vi "Port config dialog.vi"(8 "error in (no error)":errorcluster, 11 "Comm ports in":T3={"Piezo driver"="COM2", "Cam Session"="", "Arduino"="COM2"}) -> (0 "error out":errorcluster, 3 "Comm ports out":T3={"Piezo driver"="COM2", "Cam Session"="", "Arduino"="COM2"})   [LabVIEW 2020]
uses:
  Controls/Config SM states--typedef.ctl
  <vilib>/vision/driver/NI_Vision_Acquisition_Software.lvlib
  7b095cd5-608e-4c75-912f-b4dce6dcc42e.vi
  <userlib>/_OpenG.lib/error/error.llb/openg_error.lvlib
  <vilib>/userDefined/High Color/IMAQdx.ctl
  Controls/Communication ports ---typedef.ctl
panel:
  out "Image":T1(plugin-control)
  out "Test result":string
  in  "Cancel Button":bool
  in  "OK Button":bool
  in  "Test Ard":bool
  in  "Test driver":bool
  in  "Test cam":bool
  in  "Arduino":refnum<visa-resource-name>="COM5"
  in  "Cam Session":T2="cam0"
  in  "Piezo driver":refnum<visa-resource-name>="UNKNOWN"
  out "Comm ports temp":T3={"Piezo driver"="COM2", "Cam Session"="", "Arduino"="COM2"}
  out "Cancelled?":bool
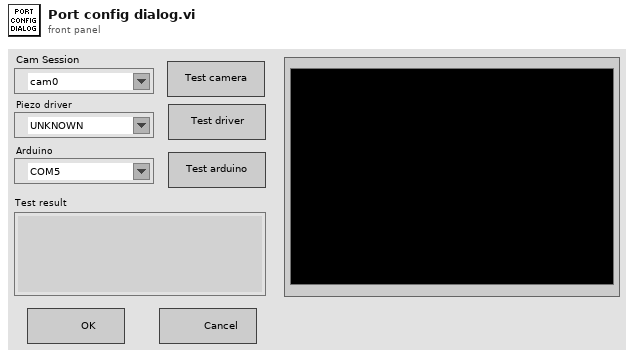
[diagram p1: front panel]
types:
  T1 = typedef "IMAQ Image.ctl" = refnum<image>
  T2 = typedef "IMAQdx.ctl" = refnum<k21>
  T3 = typedef "Communication ports ---typedef.ctl" = cluster{"Piezo driver":refnum<visa-resource-name>, "Cam Session":T2, "Arduino":refnum<visa-resource-name>}
  T4 = typedef "Config SM states--typedef.ctl" = enum16{"Init", "Wait", "Update status", "Accept", "Cancel", "Exit"}
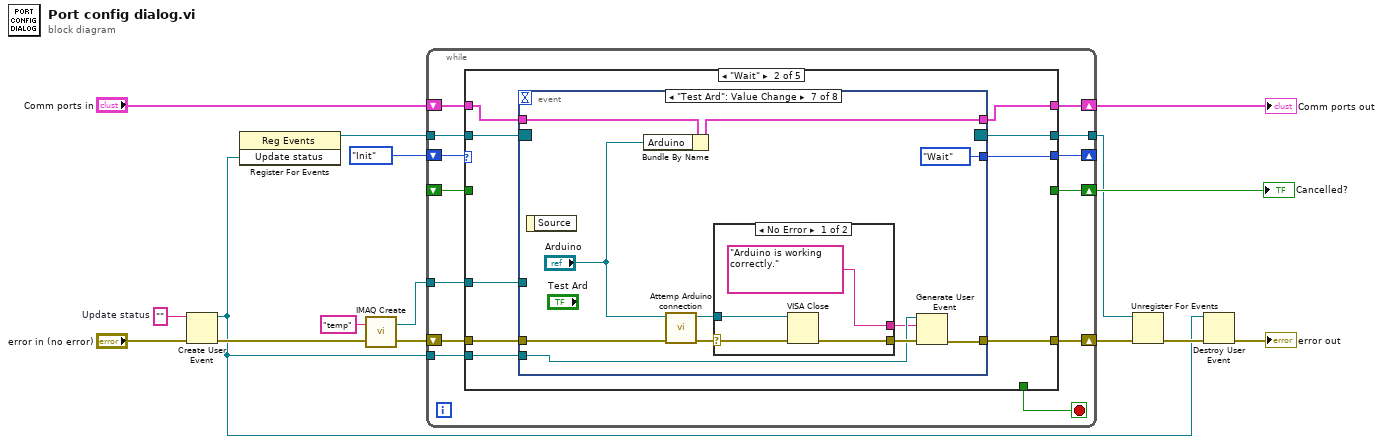
[diagram p0: block diagram]
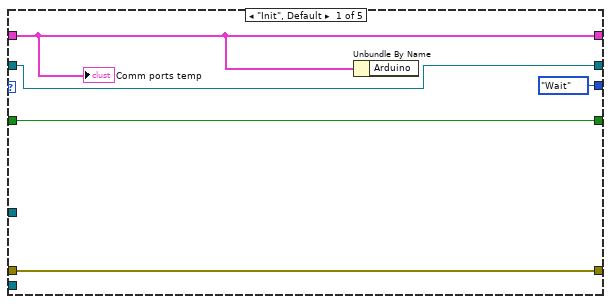
[diagram p2: hidden frame]
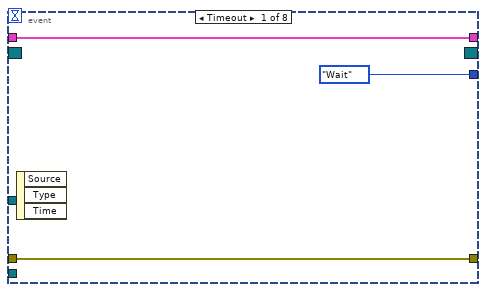
[diagram p3: hidden frame]
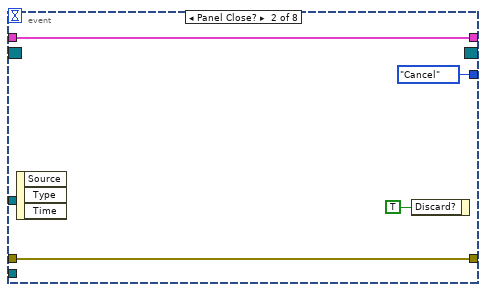
[diagram p4: hidden frame]
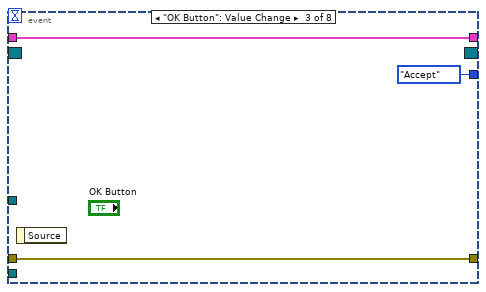
[diagram p5: hidden frame]
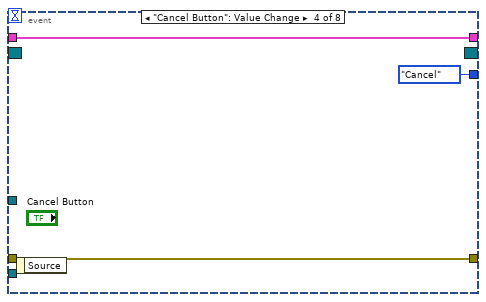
[diagram p6: hidden frame]
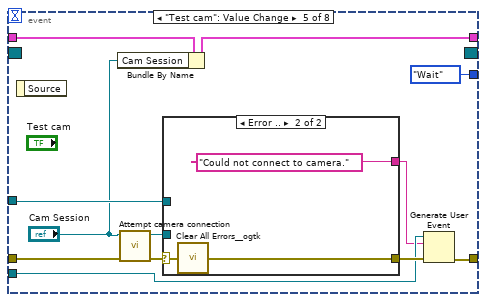
[diagram p7: hidden frame]
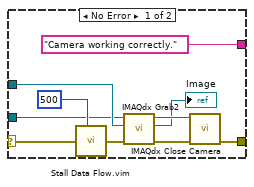
[diagram p8: hidden frame]
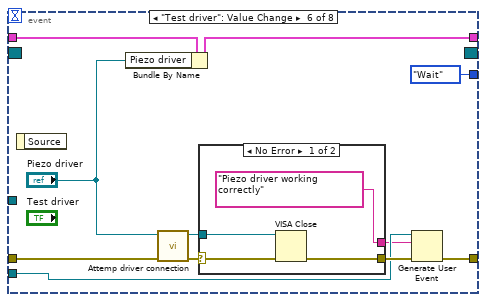
[diagram p9: hidden frame]
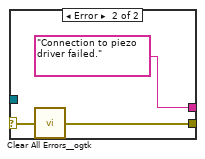
[diagram p10: hidden frame]
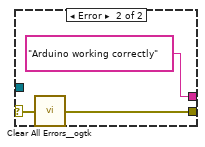
[diagram p11: hidden frame]
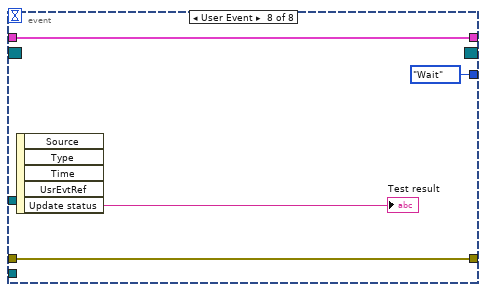
[diagram p12: hidden frame]
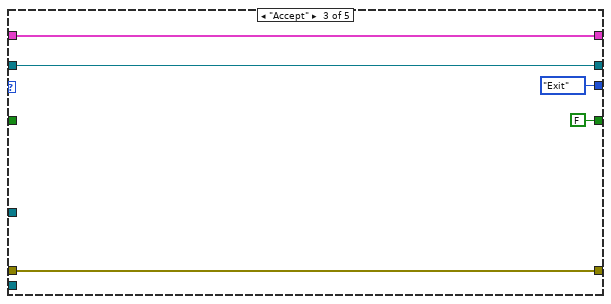
[diagram p13: hidden frame]
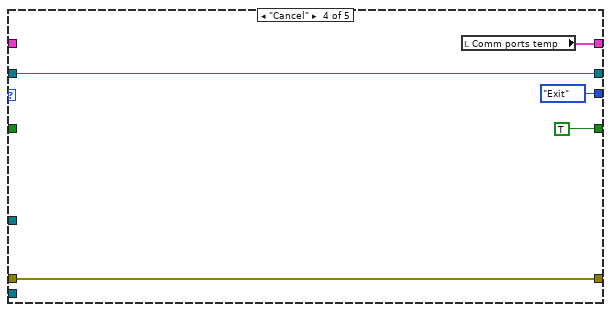
[diagram p14: hidden frame]
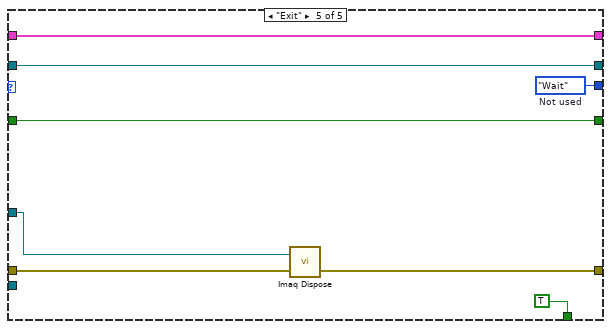
[diagram p15: hidden frame]
diagram:
  w6 = ""  # Update status
  n1 = Create User Event(user event datatype=w6, error in="error in (no error)") -> (user event=w1:refnum<user-event>, error out=w7:errorcluster)
  n2 = register-events(w1) -> (reference out=w5:refnum<event-registration>)  [unwired: 2 in, 1 out]
  n3 = call "IMAQ Create"("Image Name"="temp", "error in (no error)"=w7) -> ("New Image"=w10:T1, "error out"=w8:errorcluster)  [unwired: 3 in]
  n4 = while {
    shift-right: [w24] -> _
    shift-left: Config_SM_states--typedef."Init" -> [w25]
    shift-right: [w22] -> w12
    shift-left: _ -> [w21]
    shift-right: [w28] -> w15
    shift-left: "Comm ports in" -> [w29]
    tunnel: w10 -> [w20]
    shift-right: [w26] -> w14
    shift-left: w8 -> [w27]
    tunnel: w5 -> [w19]
    tunnel: [w18] -> w2
    tunnel: w1 -> [w17]
    stop <- w23 stop-if-true
    n5 = case shown="\"Wait\"" w25 {
      tunnel: w29 -> [w31 w40 w126 _ w139]
      tunnel: [w31 w39 w126 w128 w139] -> w28
      tunnel: w27 -> [w34 w42 w125 w131 w138]
      tunnel: [w34 w41 w125 w131 w135] -> w26
      tunnel: [Config_SM_states--typedef."Wait" w43 Config_SM_states--typedef."Exit" ("Not used") Config_SM_states--typedef."Exit" w137] -> w24
      tunnel: [_ _ _ _ TRUE] -> w23
      tunnel: [w32 _ FALSE TRUE w133] -> w22
      tunnel: w21 -> [w32 _ _ _ w133]
      tunnel: w20 -> [_ w38 _ _ w134]
      tunnel: w19 -> [w30 w37 w122 w127 w132]
      tunnel: [w30 w36 w122 w127 w132] -> w18
      tunnel: w17 -> [_ w35 _ _ _]
      frame "Init", Default {
        n6 = Unbundle By Name(w31) -> ()  [unwired: 1 out]
        "Comm ports temp" <- w31
      }
      frame "Wait" {
        n7 = event shown="[6] \"Test Ard\": Value Change" {
          selector: w37 -> [_ _ _ _ _ _ _ _]
          dyn-events: [_ _ _ _ _ _ _ _] -> w36
          timeout: _ -> [_ _ _ _ _ _ _ _]
          tunnel: [Config_SM_states--typedef."Wait" Config_SM_states--typedef."Cancel" Config_SM_states--typedef."Accept" Config_SM_states--typedef."Cancel" Config_SM_states--typedef."Wait" Config_SM_states--typedef."Wait" Config_SM_states--typedef."Wait" Config_SM_states--typedef."Wait"] -> w43
          tunnel: w42 -> [w45 w48 w53 w56 w64 w92 w108 w121]
          tunnel: [w45 w48 w53 w56 w59 w85 w103 w121] -> w41
          tunnel: w40 -> [w44 w47 w52 w55 w67 w91 w110 w120]
          tunnel: [w44 w47 w52 w55 w66 w89 w109 w120] -> w39
          tunnel: w38 -> [_ _ _ _ w65 _ _ _]
          tunnel: w35 -> [_ _ _ _ w58 w84 w102 _]
          event Timeout {
            n8 = event-data() -> ()  [unwired: 1 in, 3 out]
          }
          event Panel Close? {
            n9 = event-data() -> ()  [unwired: 1 in, 3 out]
            n10 = event-data("Discard?"=TRUE) -> ()  [unwired: 1 in, 1 out]
          }
          event "OK Button": Value Change {
            n11 = event-data() -> ()  [unwired: 1 in, 1 out]
          }
          event "Cancel Button": Value Change {
            n12 = event-data() -> ()  [unwired: 1 in, 1 out]
          }
          event "Test cam": Value Change {
            n13 = event-data() -> ()  [unwired: 1 in, 1 out]
            n14 = Bundle By Name(cluster=w67, "Cam Session"="Cam Session") -> (w66:T3)
            n15 = call "Attempt camera connection.vi"("error in (no error)"=w64, "Camera session"="Cam Session") -> ("error out"=w63:errorcluster, "Cam session Out"=w62:T2)  [unwired: 8 in]
            n16 = case shown="Error .." w63 {
              selector: w63 -> [w71 w80]
              tunnel: [w73 w81] -> w60
              tunnel: w65 -> [w72 _]
              tunnel: w62 -> [w70 _]
              tunnel: ["Camera working correctly." "Could not connect to camera."] -> w57
              frame No Error {
                n17 = call "Stall Data Flow.vim"("value in"=w71, "milliseconds to wait"=u32 500) -> ("value out"=w76:errorcluster)  [unwired: 1 out]
                n18 = call <vilib>:"IMAQdx Grab2.vi"("error in"=w76, "Image In"=w72, "Session In"=w70) -> ("error out"=w78:errorcluster, "Image Out"=→"Image":T1, "Session Out"=w77:T2)  [unwired: 5 in, 1 out]
                n19 = call <vilib>:"IMAQdx Close Camera.vi"("error in"=w78, "Session In"=w77) -> ("error out"=w73:errorcluster)  [unwired: 9 in]
              }
              frame Error {
                n20 = call <userlib>:"Clear All Errors__ogtk.vi"("Upsteam Error (optional)"=w80, "Error In"=w80) -> ("Error Out"=w81:errorcluster)  [unwired: 2 in]
              }
            }
            n21 = Generate User Event(user event=w58, event data cluster=w57, error in=w60) -> (error out=w59:errorcluster)  [unwired: 1 in, 1 out]
          }
          event "Test driver": Value Change {
            n22 = event-data() -> ()  [unwired: 1 in, 1 out]
            n23 = Bundle By Name(cluster=w91, "Piezo driver"="Piezo driver") -> (w89:T3)
            n24 = call "Attemp driver connection.vi"("error in (no error)"=w92, "COM port in"="Piezo driver") -> ("error out"=w88:errorcluster, "COM port out"=w82:refnum<visa-resource-name>)  [unwired: 8 in]
            n25 = case shown="No Error" w88 {
              selector: w88 -> [w96 w99]
              tunnel: [w94 w98] -> w87
              tunnel: ["Piezo driver working correctly" "Connection to piezo driver failed."] -> w83
              tunnel: w82 -> [w93 _]
              frame No Error {
                n26 = VISA Close(VISA resource name=w93, error in (no error)=w96) -> (error out=w94:errorcluster)
              }
              frame Error {
                n27 = call <userlib>:"Clear All Errors__ogtk.vi"("Error In"=w99) -> ("Error Out"=w98:errorcluster)  [unwired: 3 in]
              }
            }
            n28 = Generate User Event(user event=w84, event data cluster=w83, error in=w87) -> (error out=w85:errorcluster)  [unwired: 1 in, 1 out]
          }
          event "Test Ard": Value Change {
            n29 = event-data() -> ()  [unwired: 1 in, 1 out]
            n30 = Bundle By Name(cluster=w110, "Arduino"="Arduino") -> (w109:T3)
            n31 = call "Attemp Arduino connection.vi"("error in (no error)"=w108, "COM port in"="Arduino") -> ("error out"=w107:errorcluster, "COM port out"=w100:refnum<visa-resource-name>)  [unwired: 8 in]
            n32 = case shown="No Error" w107 {
              selector: w107 -> [w114 w117]
              tunnel: [w112 w116] -> w104
              tunnel: ["Arduino is working correctly." "Arduino working correctly"] -> w101
              tunnel: w100 -> [w111 _]
              frame No Error {
                n33 = VISA Close(VISA resource name=w111, error in (no error)=w114) -> (error out=w112:errorcluster)
              }
              frame Error {
                n34 = call <userlib>:"Clear All Errors__ogtk.vi"("Error In"=w117) -> ("Error Out"=w116:errorcluster)  [unwired: 3 in]
              }
            }
            n35 = Generate User Event(user event=w102, event data cluster=w101, error in=w104) -> (error out=w103:errorcluster)  [unwired: 1 in, 1 out]
          }
          event User Event {
            n36 = event-data() -> ("Update status"=→"Test result":string)  [unwired: 1 in, 4 out]
          }
        }
      }
      frame "Accept" {
      }
      frame "Cancel" {
        n37 = local read "Comm ports temp"() -> (w128:T3)
      }
      frame "Exit" {
        w137 = Config_SM_states--typedef."Wait"  # Not used
        n38 = call "Imaq Dispose"("Image"=w134, "error in (no error)"=w138) -> ("error out"=w135:errorcluster)  [unwired: 4 in]
      }
    }
  }
  "Comm ports out" <- w15
  "Cancelled?" <- w12
  n39 = Unregister For Events(event registration refnum=w2, error in=w14) -> (error out=w3:errorcluster)
  n40 = Destroy User Event(user event=w1, error in=w3) -> (error out=→"error out":errorcluster)
